vi "_Wait for Server.vi"(4 "error in":errorcluster, 5 "Timeout (8s)":u32=8000, 6 "For Ready Signal? (T)":bool=TRUE, 7 "Indicator Ref":refnum<vi>) -> (0 "error out":errorcluster)   [LabVIEW 2012]
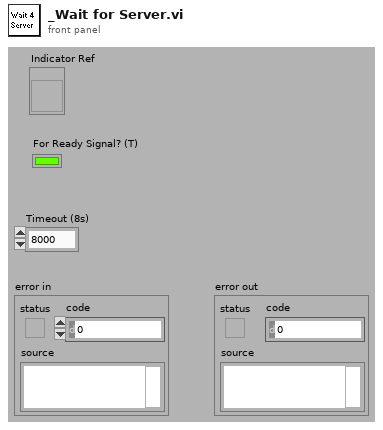
[diagram p1: front panel]
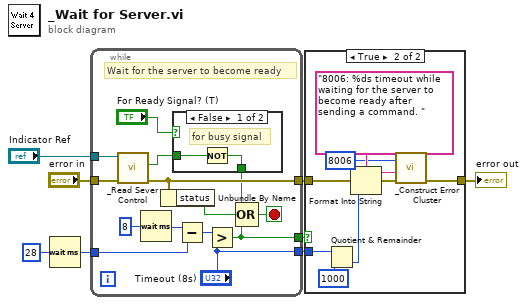
[diagram p0: block diagram]
diagram:
  n1 = Wait (ms)(milliseconds to wait=u32 28) -> (millisecond timer value=w5:u32)
  n2 = while {
    tunnel: w5 -> [w20]
    tunnel: [w14] -> w6
    tunnel: "error in" -> [w17]
    tunnel: [w15] -> w3
    tunnel: "Indicator Ref" -> [w13]
    tunnel: ["Timeout (8s)"] -> w1
    stop <- w18 stop-if-true
    # "Wait for the server to become ready"
    n3 = call "_Read Sever Control.vi"("error in (no error)"=w17, "Control Ref"=w13) -> ("error out"=w14:errorcluster, "Boolean"=w11:bool)  [unwired: 2 in, 2 out]
    n4 = Wait (ms)(milliseconds to wait=u32 8) -> (millisecond timer value=w21:u32)
    n5 = Unbundle By Name(w14) -> ("status"=w16:bool)
    n6 = case shown="False" "For Ready Signal? (T)" {
      tunnel: [w23 w25] -> w10
      tunnel: w11 -> [w24 w25]
      frame False {
        # "for busy signal"
        n7 = Not(x=w24) -> (.not. x?=w23:bool)
      }
      frame True {
      }
    }
    n8 = Subtract(x=w21, y=w20) -> (x-y=w19:u32)
    n9 = Greater?(x=w19, y="Timeout (8s)") -> (0:w15:bool)
    n10 = Compound Arithmetic op=OR(w10, w16, w15) -> (w18:bool)
  }
  n11 = case shown="True" w3 {
    tunnel: w6 -> [w26 w34]
    tunnel: [w26 w33] -> w7
    tunnel: w1 -> [_ w30]
    frame False {
    }
    frame True {
      n12 = Quotient & Remainder(x=w30, y=u32 1000) -> (floor(x/y)=w29:u32)  [unwired: 1 out]
      n13 = Format Into String(format string="8006: %ds timeout while waiting for the server to become ready after sending a command. " ("f"), w29) -> (resulting string=w31:string)  [unwired: 2 in, 1 out]
      n14 = call "_Construct Error Cluster.vi"("error in"=w34, "reason"=w31, "errorCode"=8006) -> ("error out"=w33:errorcluster)  [unwired: 1 in, 3 out]
    }
  }
  "error out" <- w7
